vi "Is True.vi"(11 "Expression in":T1) -> (3 "Is True?":bool)   [LabVIEW 2020]
uses:
  ExpressionType.ctl
  Expression.ctl
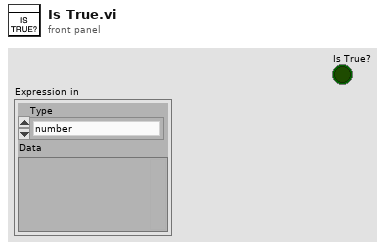
[diagram p1: front panel]
types:
  T1 = typedef "Expression.ctl" = cluster{"Type":T2, "Data":variant}
  T2 = typedef "ExpressionType.ctl" = enum16{"number", "string", "symbol", "primitive", "list", "closure", "macro", "nil", "error"}
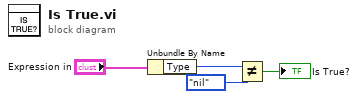
[diagram p0: block diagram]
diagram:
  n1 = Unbundle By Name("Expression in") -> ("Type"=w3:T2)
  n2 = Not Equal?(x=w3, y=ExpressionType."nil") -> (x != y?=→"Is True?":bool)
